vi "niFPGA Backlash_m.vi"   [LabVIEW 2017]
doc: "Implements a backlash or deadband function. <B>output</B> does not change until <B>input</B> differs from the previous <B>output</B> by at least half of <B>deadband</B>. The data type you wire to <B>input</B> determines the <B>output</B> data type."
uses:
  <vilib>/rvi/Analysis/common/FxpNativeNode/niFpgaFxpNative.xnode
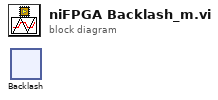
[diagram p0: block diagram]
diagram:
  n1 = xnode "Backlash"() -> ()  [unwired: 4 in, 1 out]
